vi "reload MathCAD.vi"(8 "error in":errorcluster, 11 "reload":bool) -> (0 "error out":errorcluster)   [LabVIEW 2015]
uses:
  mathcad/Simple/MathCAD cmd.ctl
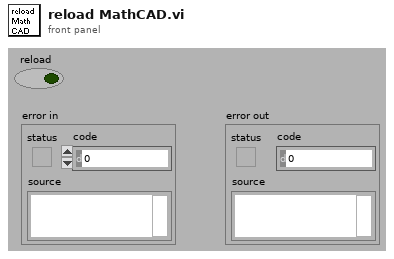
[diagram p1: front panel]
types:
  T1 = typedef "MathCAD cmd.ctl" = enum16{"Open App", "Open Worksheet", "Close Worksheet", "Load Variable Ref", "Send Number", "Send Cluster", "Send Array", "Send String", "Calculate", "Get MathCAD data", "Close MathCAD"}
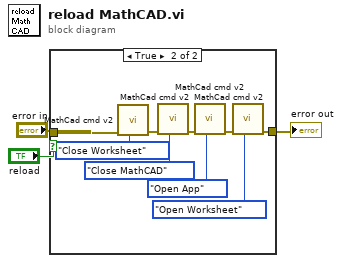
[diagram p0: block diagram]
diagram:
  n1 = case shown="True" "reload" {
    tunnel: [w4 w12] -> w3
    tunnel: "error in" -> [w4 w8]
    frame False {
    }
    frame True {
      n2 = call "MathCad cmd v2.vi"("MathCAD cmds"=MathCAD_cmd."Close Worksheet", "error in"=w8) -> ("first error out"=w9:errorcluster)  [unwired: 8 in, 1 out]
      n3 = call "MathCad cmd v2.vi"("MathCAD cmds"=MathCAD_cmd."Close MathCAD", "error in"=w9) -> ("first error out"=w5:errorcluster)  [unwired: 8 in, 1 out]
      n4 = call "MathCad cmd v2.vi"("MathCAD cmds"=MathCAD_cmd."Open App", "error in"=w5) -> ("first error out"=w11:errorcluster)  [unwired: 8 in, 1 out]
      n5 = call "MathCad cmd v2.vi"("MathCAD cmds"=MathCAD_cmd."Open Worksheet", "error in"=w11) -> ("first error out"=w12:errorcluster)  [unwired: 8 in, 1 out]
    }
  }
  "error out" <- w3
